vi "Open_Door.vi"(8 "error in (no error)":errorcluster caption="entrée d'erreur (pas d'erreur)", 11 "Class Shielding_ Box en entrée":refnum<class "Class Shielding_ Box JC-PB3044.lvclass">) -> (0 "error out":errorcluster caption="sortie d'erreur", 3 "Class Shielding_ Box en sortie":refnum<class "Class Shielding_ Box JC-PB3044.lvclass">)   [LabVIEW 2020, in "Library Instrument & Equipement.lvlib" / "Library Shielding box.lvlib" / "Class Shielding_ Box JC-PB3044.lvclass"]
uses:
  Class Shielding_ Box JC-PB3044.lvclass
  C:/Users/ngarcin/OneDrive - Altyor/Standard TB/Class/Shielding box/Class Shielding box (Default)/Class Shielding_ Box (Default).lvclass
  Class Shielding_ Box JC-PB3044.lvclass/Class Shielding_ Box JC-PB3044.ctl
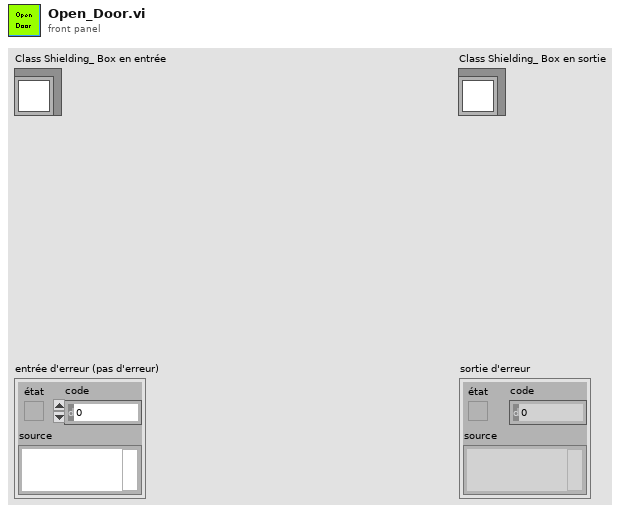
[diagram p1: front panel]
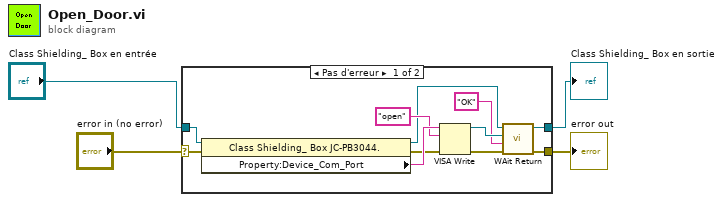
[diagram p0: block diagram]
diagram:
  n1 = case shown="Pas d'erreur" "error in (no error)" {
    selector: "error in (no error)" -> [w12 w17]
    tunnel: [w8 w17] -> w2
    tunnel: [w6 w16] -> w1
    tunnel: "Class Shielding_ Box en entrée" -> [w15 w16]
    frame No Error {
      n2 = property class="Class Shielding_ Box JC-PB3044."(reference=w15, error in=w12) -> (reference out=w7:refnum<class "Class Shielding_ Box JC-PB3044.lvclass">, error out=w11:errorcluster, "Property:Device_Com_Port"=w14:string)
      n3 = VISA Write(VISA resource name=w14, write buffer="open" ("buffer d'écriture"), error in (no error)=w11) -> (VISA resource name out=w10:refnum<visa-resource-name>, error out=w9:errorcluster)  [unwired: 1 out]
      n4 = call "WAit Return.vi"("entrée d'erreur (pas d'erreur)"=w9, "String Wait"="OK", "VISA resource name"=w10, "Class Shielding_ Box JC-PB3044 en entrée"=w7) -> ("sortie d'erreur"=w8:errorcluster, "Class Shielding_ Box JC-PB3044 en sortie"=w6:refnum<class "Class Shielding_ Box JC-PB3044.lvclass">)  [unwired: 5 in, 1 out]
    }
    frame Error {
    }
  }
  "error out" <- w2
  "Class Shielding_ Box en sortie" <- w1
